vi "Get Slide Count.vi"(8 "error in (no error)":errorcluster, 11 "Parse Presentation in":refnum<class "Parse Presentation.lvclass">) -> (0 "error out":errorcluster, 3 "Parse Presentation out":refnum<class "Parse Presentation.lvclass">)   [LabVIEW 2015, in "Parse Presentation.lvclass"]
uses:
  Parse Presentation.lvclass
  Parse Presentation.lvclass/Parse Presentation.ctl
  D:/Metis Automation/ppt-parsing/CSharp/ParsePpt/ParsePpt/bin/Debug/ParsePpt.dll
  CSharp/ParsePpt/ParsePpt/bin/Debug/ParsePpt.dll
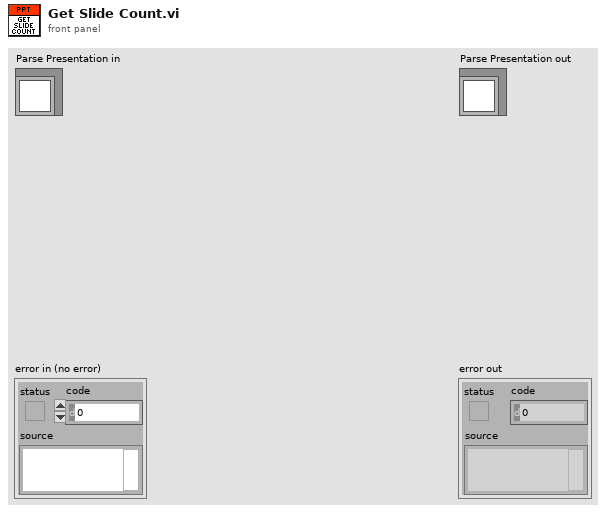
[diagram p1: front panel]
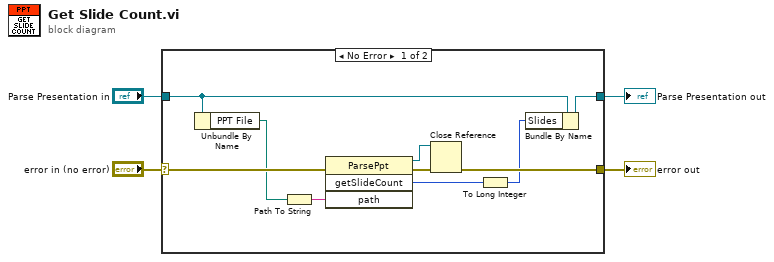
[diagram p0: block diagram]
diagram:
  n1 = case shown="No Error" "error in (no error)" {
    selector: "error in (no error)" -> [w13 w16]
    tunnel: [w9 w16] -> w3
    tunnel: [w7 w15] -> w1
    tunnel: "Parse Presentation in" -> [w14 w15]
    frame No Error {
      n2 = Unbundle By Name(w14) -> ("PPT File"=w10:path)
      n3 = Path To String(path=w10) -> (string=w11:string)
      n4 = invoke class="ParsePpt" method="getSlideCount"(error in=w13, "path"=w11) -> (reference out=w8:refnum<k24>, error out=w12:errorcluster, "getSlideCount"=w6:i64)  [unwired: 2 in, 1 out]
      n5 = Close Reference(reference=w8, error in (no error)=w12) -> (error out=w9:errorcluster)
      n6 = To Long Integer(number=w6) -> (32bit integer=w5:i32)
      n7 = Bundle By Name(cluster=w14, "Slides"=w5) -> (w7:refnum<class "Parse Presentation.lvclass">)
    }
    frame Error {
    }
  }
  "error out" <- w3
  "Parse Presentation out" <- w1
